vi "Save-temperature.vi"(8 "error in":errorcluster, 10 "Storage element in":T1 {"Temperature characteristics"."Stand. dev. temperature" format="%#.1f"; "Temperature characteristics"."Min. temperature" format="%#.0f"; "Temperature characteristics"."Max. temperature" format="%#.0f"; "Temperature characteristics"."Average temperature" format="%#.0f"}, 11 "Storage params. ref. in":refnum<data-value>) -> (0 "error IO":errorcluster, 2 "Storage element":T1 {"Temperature characteristics"."Stand. dev. temperature" format="%#.1f"; "Temperature characteristics"."Min. temperature" format="%#.0f"; "Temperature characteristics"."Max. temperature" format="%#.0f"; "Temperature characteristics"."Average temperature" format="%#.0f"}, 3 "Storage params. ref.":refnum<data-value>)   [LabVIEW 2013, in "CameraVision.lvlib" / "CV-Main.lvclass"]
uses:
  CV-Main.lvclass
  Storage/CV-Storage.lvclass
  Buffers/Storage-buffer.ctl
  <vilib>/vision/Image Controls.llb/IMAQ Image.ctl
  Temperature/Temperature-characteristics.ctl
  Analysis/Characteristics-cluster.ctl
  Storage/CV-Storage.lvclass/CV-Storage.ctl
  Storage/Read Temperature file reference W.vi
  Storage/Read Save what.vi
  Storage/Read CharacteristicsTemperature headers.vi
  Temperature/CV-Temperature.lvclass
  Analysis/CV-Analysis.lvclass
  Buffers/CV-Buffers.lvclass
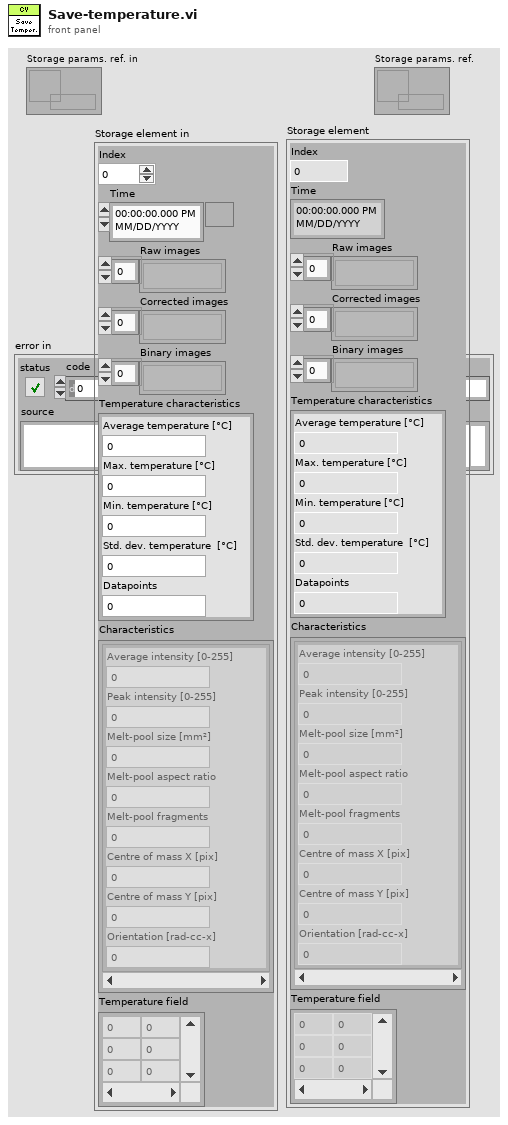
[diagram p1: front panel]
types:
  T1 = typedef "CameraVision.lvlib/CV-Buffers.lvclass/Storage-buffer.ctl" = cluster{"Index":i32, "Time":timestamp, "Raw images":T2[], "Corrected images":T2[], "Binary images":T2[], "Temperature characteristics":T3, "Characteristics":T4[], "Temperature field":dbl[][]}
  T2 = typedef "IMAQ Image.ctl" = refnum<image>
  T3 = typedef "CameraVision.lvlib/CV-Temperature.lvclass/Temperature-characteristics.ctl" = cluster{"Average temperature ":dbl, "Max. temperature":dbl, "Min. temperature":dbl, "Stand. dev. temperature":dbl, "Datapoints":dbl}
  T4 = typedef "CameraVision.lvlib/CV-Analysis.lvclass/Characteristics-cluster.ctl" = cluster{"Average intensity":dbl, "Peak intensity":dbl, "Melt-pool size":dbl, "Melt-pool aspect ratio":dbl, "Melt-pool fragments":dbl, "Centre of mass X":dbl, "Centre of mass Y":dbl, "Orientation":dbl}
  T5 = cluster{"Original":bool, "Corrected":bool, "Binary":bool, "Temperature":bool, "Characteristics":bool, "Mapping":bool, "TemperatureValues":bool}
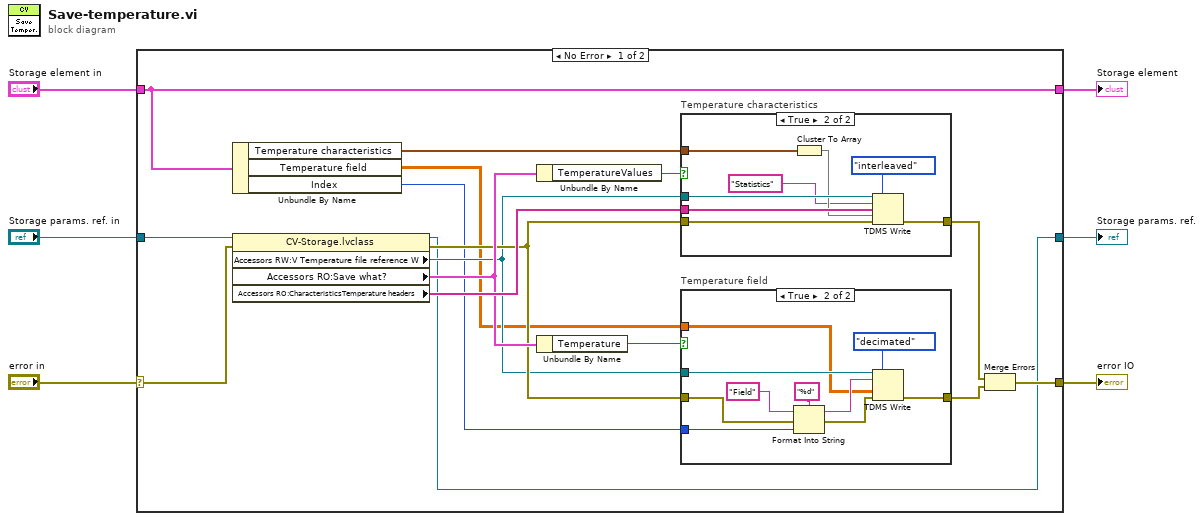
[diagram p0: block diagram]
diagram:
  n1 = case shown="No Error" "error in" {
    selector: "error in" -> [w21 w45]
    tunnel: [w8 w45] -> w6
    tunnel: "Storage params. ref. in" -> [w22 w44]
    tunnel: "Storage element in" -> [w9 w43]
    tunnel: [w7 w44] -> w2
    tunnel: [w9 w43] -> w1
    frame No Error {
      n2 = Unbundle By Name(w9) -> ("Temperature characteristics"=w15:T3, "Temperature field"=w16:dbl[][], "Index"=w14:i32)
      n3 = property class="CV-Storage.lvclass"(reference=w22, error in=w21) -> (reference out=w7:refnum<data-value>, error out=w18:errorcluster, "Accessors RW:V Temperature file reference W"=w17:refnum<k34>, "Accessors RO:Save what?"=w19:T5, "Accessors RO:CharacteristicsTemperature headers"=w20:string[])
      n4 = Unbundle By Name(w19) -> ("TemperatureValues"=w13:bool)
      n5 = Unbundle By Name(w19) -> ("Temperature"=w12:bool)
      n6 = case "Temperature characteristics" shown="True" w13 {
        tunnel: w15 -> [_ w36]
        tunnel: w17 -> [_ w42]
        tunnel: w20 -> [_ w41]
        tunnel: w18 -> [w34 w35]
        tunnel: [w34 w40] -> w11
        frame False {
        }
        frame True {
          n7 = Cluster To Array(cluster=w36) -> (array=w39:dbl[])
          n8 = TDMS Write(0:w42, 1:enum16{"decimated", "interleaved"}."interleaved" ("data layout (0:decimated)"), 5:"Statistics" ("group name in (Untitled)"), 7:w41, 9:w39, 11:w35) -> (15:w40:errorcluster)  [unwired: 3 out]
        }
      }
      n9 = case "Temperature field" shown="True" w12 {
        tunnel: w16 -> [_ w24]
        tunnel: w17 -> [_ w33]
        tunnel: w18 -> [w23 w25]
        tunnel: [w23 w32] -> w10
        tunnel: w14 -> [_ w26]
        frame False {
        }
        frame True {
          n10 = Format Into String(format string="%d", initial string="Field", error in=w25, w26) -> (resulting string=w27:string, error out=w29:errorcluster)
          n11 = TDMS Write(0:w33, 1:enum16{"decimated", "interleaved"}."decimated" ("data layout (0:decimated)"), 5:w27, 9:w24, 11:w29) -> (15:w32:errorcluster)  [unwired: 1 in, 3 out]
        }
      }
      n12 = Merge Errors(w11, w10) -> (w8:errorcluster)
    }
    frame Error {
    }
  }
  "error IO" <- w6
  "Storage params. ref." <- w2
  "Storage element" <- w1
